vi "SNR.vi"(1 "Signal with Noise":dbl[](array[numeric]) format="%#_13g", 2 "Clear":dbl[](array[numeric]) format="%#_13g") -> (0 "SNR":dbl format="%#_13g")   [LabVIEW 2014]
uses:
  <vilib>/Analysis/5stat.llb/RMS (DBL).vi
  <vilib>/Analysis/NI_AALPro.lvlib
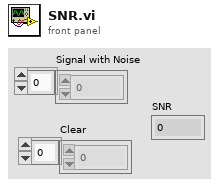
[diagram p1: front panel]
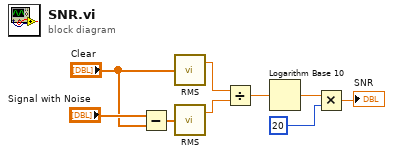
[diagram p0: block diagram]
diagram:
  n1 = Subtract(x="Signal with Noise", y="Clear") -> (x-y=w5:dbl[])
  n2 = call-poly <vilib>:"RMS.vi"("X"="Clear") -> ("rms value"=w2:dbl)  [unwired: 1 out]
  n3 = call-poly <vilib>:"RMS.vi"("X"=w5) -> ("rms value"=w1:dbl)  [unwired: 1 out]
  n4 = Divide(x=w2, y=w1) -> (x/y=w3:dbl)
  n5 = Logarithm Base 10(1:w3) -> (0:w8:dbl)
  n6 = Multiply(x=w8, y=20) -> (x*y=→"SNR":dbl)
